vi "Exercise 3.3 Applying What I've Learned.vi"() -> ()   [LabVIEW 2012]
uses:
  <vilib>/express/express analysis/Spectral/Block/exnSpectralBlock spectral measurements RMS poly.vi
  <vilib>/express/express analysis/Spectral/Block/exnSpectralBlock spectral measurements RMS DDT.vi
  <vilib>/express/express analysis/Spectral/XNode/ExpressSpectralMeasurementsBlockNode.xnode
panel:
  out "Fast Fourier Transform Signal":dynamicdata(graph)
  out "Filtered Signal Chart":dynamicdata(graph)
  in  "stop":bool
  in  "Control Frequency":dbl
  out "Unfiltered Signal":dynamicdata(graph)
  out "Filtered Signal":dynamicdata(graph)
  out "Boolean":bool
  in  "Cut Off Frequency":dbl
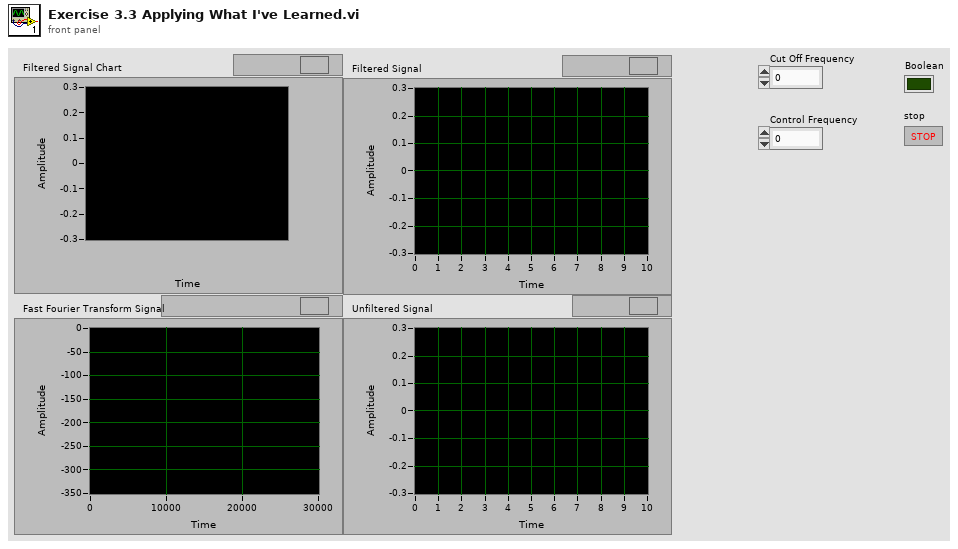
[diagram p1: front panel]
types:
  T1 = cluster{"averaging mode":u16, "weighting mode":u16, "number of averages":u32}
  T2 = cluster{"dB On (F)":bool, "unwrap phase (F)":bool, "convert to degree (F)":bool}
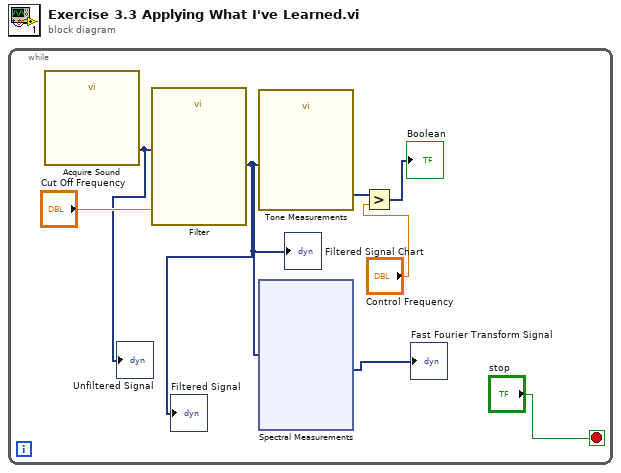
[diagram p0: block diagram]
diagram:
  n1 = while {
    stop <- "stop" stop-if-true
    n2 = call "Acquire Sound"() -> ("Data"=w5:dynamicdata)  [unwired: 18 in, 1 out]
    "Unfiltered Signal" <- w5
    n3 = call "Filter"("Lower Cut-Off"="Cut Off Frequency", "Signal"=w5) -> ("Filtered Signal"=w2:dynamicdata)  [unwired: 8 in, 1 out]
    "Filtered Signal" <- w2
    "Filtered Signal Chart" <- w2
    n4 = call "Tone Measurements"("Signals"=w2) -> ("Frequency"=w7:dynamicdata)  [unwired: 8 in, 2 out]
    n5 = xnode "Spectral Measurements"("Signals"=w2) -> ("FFT - (RMS)"=→"Fast Fourier Transform Signal":dynamicdata)  [unwired: 1 in, 2 out]
    n6 = Greater?(x=w7, y="Control Frequency") -> (0:→"Boolean":dynamicdata)
  }
